vi "RC_CHANNELS_OVERRIDE.vi"(11 "Payload":T1) -> (3 "MAVLink Message":u8[](array[numeric]))   [LabVIEW 2014]
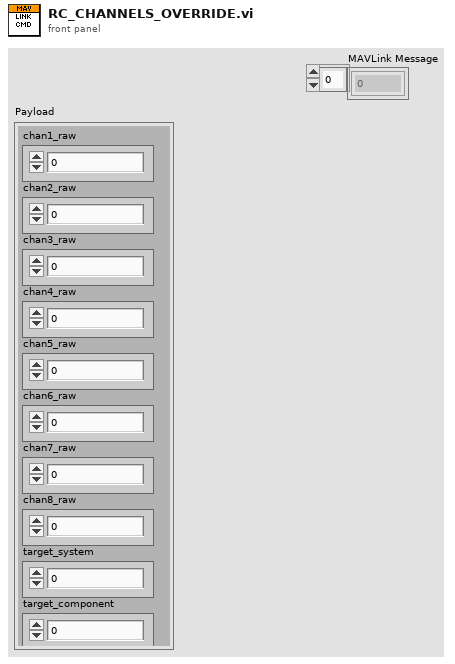
[diagram p1: front panel]
types:
  T1 = cluster{"chan1_raw":u16, "chan2_raw":u16, "chan3_raw":u16, "chan4_raw":u16, "chan5_raw":u16, "chan6_raw":u16, "chan7_raw":u16, "chan8_raw":u16, "target_system":u8, "target_component":u8}
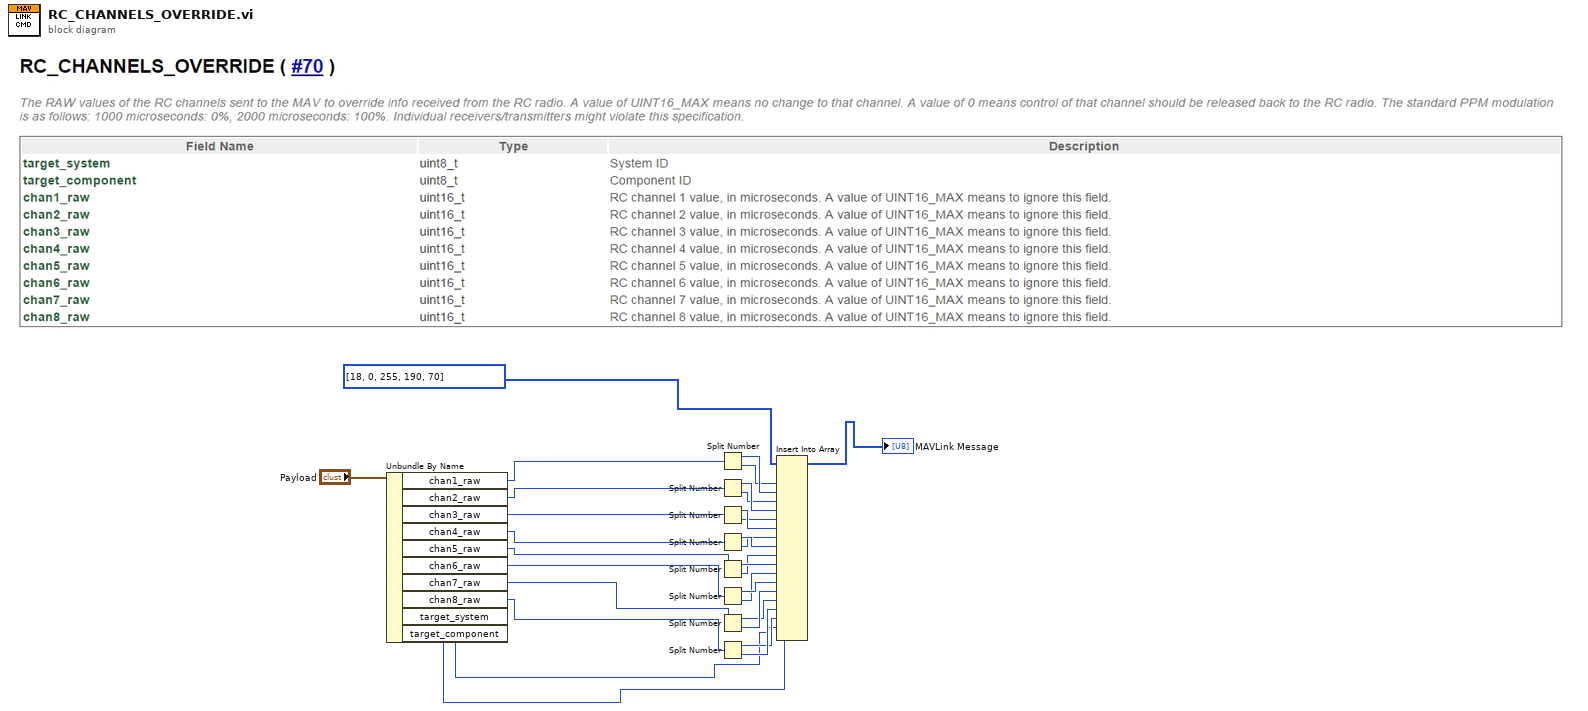
[diagram p0: block diagram]
diagram:
  n1 = Unbundle By Name("Payload") -> ("chan1_raw"=w26:u16, "chan2_raw"=w23:u16, "chan3_raw"=w20:u16, "chan4_raw"=w17:u16, "chan5_raw"=w14:u16, "chan6_raw"=w11:u16, "chan7_raw"=w7:u16, "chan8_raw"=w4:u16, "target_system"=w3:u8, "target_component"=w2:u8)
  n2 = Split Number(x=w26) -> (hi(x)=w28:u8, lo(x)=w25:u8)
  n3 = Split Number(x=w23) -> (hi(x)=w24:u8, lo(x)=w22:u8)
  n4 = Split Number(x=w20) -> (hi(x)=w21:u8, lo(x)=w19:u8)
  n5 = Split Number(x=w17) -> (hi(x)=w18:u8, lo(x)=w16:u8)
  n6 = Split Number(x=w14) -> (hi(x)=w15:u8, lo(x)=w13:u8)
  n7 = Split Number(x=w11) -> (hi(x)=w12:u8, lo(x)=w10:u8)
  n8 = Split Number(x=w7) -> (hi(x)=w8:u8, lo(x)=w9:u8)
  n9 = Split Number(x=w4) -> (hi(x)=w5:u8, lo(x)=w6:u8)
  n10 = Insert Into Array(array=u8[] [18, 0, 255, 190, 70], new element #1=w25, new element #2=w28, new element #3=w22, new element #4=w24, new element #5=w19, new element #6=w21, new element #7=w16, new element #8=w18, new element #9=w13, new element #10=w15, new element #11=w10, new element #12=w12, new element #13=w9, new element #14=w8, new element #15=w6, new element #16=w5, new element #17=w3, new element #18=w2) -> (→"MAVLink Message":u8[])  [unwired: 1 in]
